vi "PV ActiveLine config relay.vi"(8 "error in (no error)":errorcluster, 9 "PV ActiveLine config relay - Cluster":T1={"Parameter"=enum." Configuration Relais 1 (045)", "Parameter\nread only<->describe"=FALSE, "Configuration R1 .. R6"=9} {"Configuration R1 .. R6" items=["0 = rot. speed switch point attained", "1 = no error", "2 = error", "3 = warning", "4 = error and/or warning", "5 = set speed attained", "6 = pump on", "7 = pump accelerates", "8 = pump decelerater", "9 = always 0 (off)", "10 = always 1 (on)", "11 = remote priority active", "12 = heating", "13 = backing pump", "14 = sealing gas", "15 = pumping station", "16 = pump rotates", "17 = pump does not rotate", "18 = TMS temperature engaged  ", "19 = Pressure below pressure switchpoint 1", "20 = Pressure below pressure switchpoint 2", "21 = Pressure below pressure switchpoint 3", "22 = Pressure below pressure switchpoint 4", "23 = Pressure below pressure switchpoint 5", "24 = Pressure below pressure switchpoint 6"]}, 10 "Adress of unit":u16=10 max=999 step=1, 11 "VISA session":refnum<visa-resource-name>) -> (0 "error out":errorcluster, 2 "response (data)":string, 3 "dup VISA session":refnum<visa-resource-name>)   [LabVIEW 2021, in "Pfeiffer Vacuum.lvlib"]
doc: "There are 6 parameters available, only one of which can be enabled at a time. \n\n Configuration Relais 1 (045)\n Configuration Relais 2 (046)\n Configuration Relais 3 (047)\n Configuration Relais 4 (048)\n Configuration Relais 5 (066)\n Configuration Relais 6 (067)\n \nNote: Any settings for an parameter that is not selected will be ignored. If a value is out of range, it will be changed to either the upper or the lower limit of the range."
uses:
  <instrlib>/Pfeiffer Vacuum/Pfeiffer Vacuum.lvlib
  <instrlib>/Pfeiffer Vacuum/Public/ActiveLine/PV ActiveLine config relay - Cluster.ctl
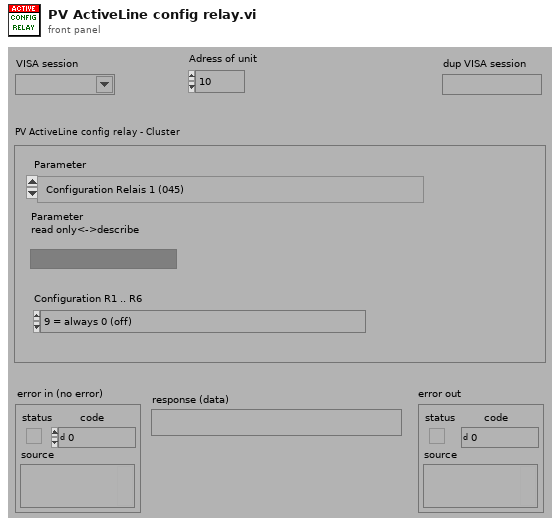
[diagram p1: front panel]
types:
  T1 = typedef "Pfeiffer Vacuum.lvlib/PV ActiveLine config relay - Cluster.ctl" = cluster{"Parameter":enum16{" Configuration Relais 1 (045)", " Configuration Relais 2 (046)", " Configuration Relais 3 (047)", " Configuration Relais 4 (048)", " Configuration Relais 5 (066)", " Configuration Relais 6 (067)"}, "Parameter\nread only<->describe":bool, "Configuration R1 .. R6":u16}
  T2 = enum16{" Configuration Relais 1 (045)", " Configuration Relais 2 (046)", " Configuration Relais 3 (047)", " Configuration Relais 4 (048)", " Configuration Relais 5 (066)", " Configuration Relais 6 (067)"}
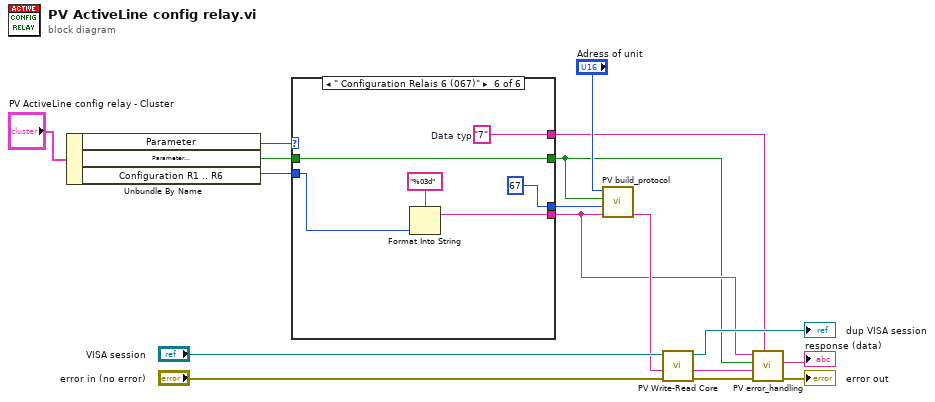
[diagram p0: block diagram]
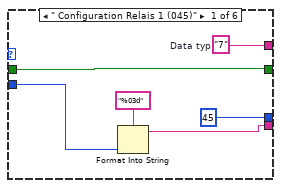
[diagram p2: hidden frame]
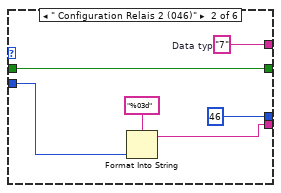
[diagram p3: hidden frame]
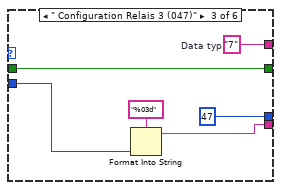
[diagram p4: hidden frame]
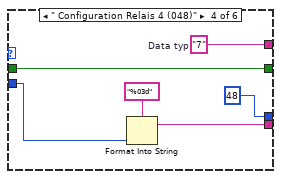
[diagram p5: hidden frame]
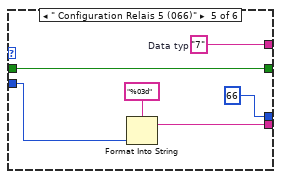
[diagram p6: hidden frame]
diagram:
  n1 = Unbundle By Name("PV ActiveLine config relay - Cluster") -> ("Parameter"=w4:T2, "Parameter\nread only<->describe"=w3:bool, "Configuration R1 .. R6"=w2:u16)
  n2 = case shown="\" Configuration Relais 6 (067)\"" w4 {
    tunnel: [u16 45 ("Parameter-number") u16 46 ("Parameter-number") u16 47 ("Parameter-number") u16 48 ("Parameter-number") u16 66 ("Parameter-number") u16 67 ("Parameter-number")] -> w16
    tunnel: [w18 w25 w34 w38 w44 w50] -> w7
    tunnel: [w21 w27 w30 w37 w43 w49] -> w6
    tunnel: [w22 w28 w32 w40 w46 w52] -> w8
    tunnel: w3 -> [w21 w27 w30 w37 w43 w49]
    tunnel: w2 -> [w19 w24 w31 w36 w42 w48]
    frame " Configuration Relais 1 (045)" {
      w22 = "7"  # Data typ
      n3 = Format Into String(format string="%03d" ("Format-String"), w19) -> (resulting string=w18:string)  [unwired: 2 in, 1 out]
    }
    frame " Configuration Relais 2 (046)" {
      w28 = "7"  # Data typ
      n4 = Format Into String(format string="%03d" ("Format-String"), w24) -> (resulting string=w25:string)  [unwired: 2 in, 1 out]
    }
    frame " Configuration Relais 3 (047)" {
      w32 = "7"  # Data typ
      n5 = Format Into String(format string="%03d" ("Format-String"), w31) -> (resulting string=w34:string)  [unwired: 2 in, 1 out]
    }
    frame " Configuration Relais 4 (048)" {
      w40 = "7"  # Data typ
      n6 = Format Into String(format string="%03d" ("Format-String"), w36) -> (resulting string=w38:string)  [unwired: 2 in, 1 out]
    }
    frame " Configuration Relais 5 (066)" {
      w46 = "7"  # Data typ
      n7 = Format Into String(format string="%03d" ("Format-String"), w42) -> (resulting string=w44:string)  [unwired: 2 in, 1 out]
    }
    frame " Configuration Relais 6 (067)" {
      w52 = "7"  # Data typ
      n8 = Format Into String(format string="%03d" ("Format-String"), w48) -> (resulting string=w50:string)  [unwired: 2 in, 1 out]
    }
  }
  n9 = call <instrlib>:"PV build_protocol.vi"("Data"=w7, "Parameter-number"=w16, "parameter\nread<->describe"=w6, "Adress"="Adress of unit") -> ("output"=w12:string)  [unwired: 3 in]
  n10 = call <instrlib>:"PV Write-Read Core.vi"("error in"="error in (no error)", "Write data in"=w12, "VISA session"="VISA session") -> ("error out"=w9:errorcluster, "response (data) out"=w10:string, "dup VISA session"=→"dup VISA session":refnum<visa-resource-name>)  [unwired: 2 in]
  n11 = call <instrlib>:"PV error_handling.vi"("Data Typ in"=w8, "error in"=w9, "response (data) in"=w10, "Parameter\nread only<->describe"=w6, "data in"=w7) -> ("error out"=→"error out":errorcluster, "Data out"=→"response (data)":string)  [unwired: 4 in, 1 out]
